vi "global_bool.vi"() -> ()   [LabVIEW 2011]
panel:
  out "rebuffering":bool
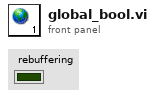
[diagram p1: front panel]
diagram:
